vi "Set Channel.vi"(0 "TCS.lvclass in":refnum<class "TCS.lvclass">, 5 "Channel":u8, 7 "I&R In":T1 {"Current" min=0.0}, 11 "error in (no error)":errorcluster) -> (4 "TCS.lvclass out":refnum<class "TCS.lvclass">, 15 "error out":errorcluster)   [LabVIEW 2016, in "TCS.lvclass"]
uses:
  Lib.llb/TCS.lvclass
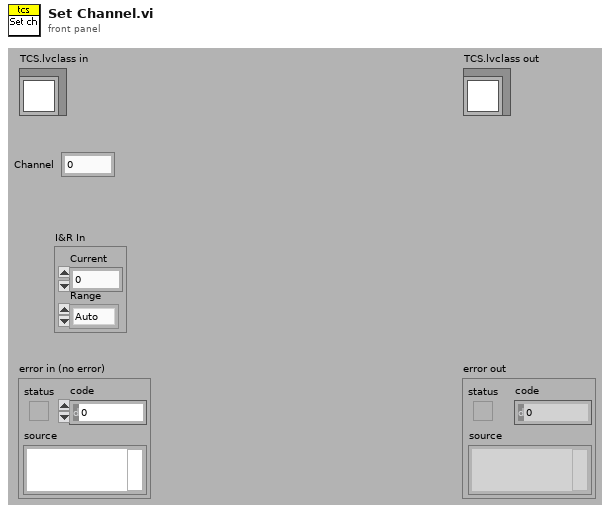
[diagram p1: front panel]
types:
  T1 = cluster{"Current":dbl, "Range":enum8{"Auto", "x1 uA", "x10 uA", "x100 uA", "x1 mA"}}
  T2 = enum8{"Auto", "x1 uA", "x10 uA", "x100 uA", "x1 mA"}
  T3 = cluster{"error":bool, "code":i32, "source":string}
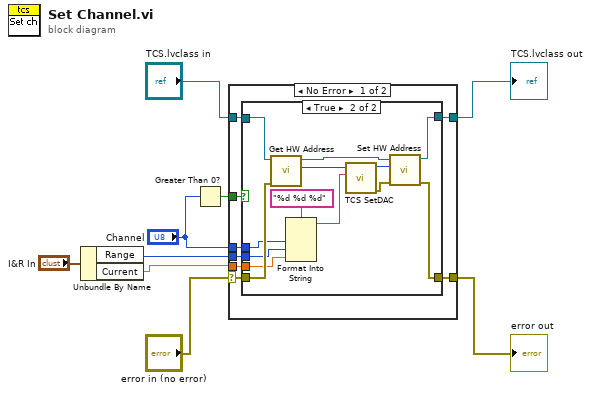
[diagram p0: block diagram]
diagram:
  n1 = Unbundle By Name("I&R In") -> ("Range"=w2:T2, "Current"=w1:dbl)
  n2 = Greater Than 0?(x="Channel") -> (x > 0?=w5:bool)
  n3 = case shown="No Error" "error in (no error)" {
    selector: "error in (no error)" -> [w17 w34]
    tunnel: "TCS.lvclass in" -> [w14 w33]
    tunnel: [w15 w33] -> w8
    tunnel: "Channel" -> [w13 _]
    tunnel: w2 -> [w12 _]
    tunnel: w1 -> [w11 _]
    tunnel: [w16 w34] -> w7
    tunnel: w5 -> [w10 _]
    frame No Error {
      n4 = case shown="True" w10 {
        tunnel: w17 -> [w19 w32]
        tunnel: [w19 w31] -> w16
        tunnel: [w18 w30] -> w15
        tunnel: w14 -> [w18 w29]
        tunnel: w13 -> [_ w23]
        tunnel: w12 -> [_ w22]
        tunnel: w11 -> [_ w21]
        frame False {
          # "Ignore Channel 0"
        }
        frame True {
          n5 = call-dynamic "Get HW Address.vi"("error in (no error)"=w32, "CS.lvclass in"=w29) -> ("HW Address"=w28:i32, "CS.lvclass out"=w20:refnum<class "TCS.lvclass">)  [unwired: 7 in, 1 out]
          n6 = Format Into String(format string="%d %d %d", w23, w22, w21) -> (resulting string=w24:string)  [unwired: 2 in, 1 out]
          n7 = call "TCS SetDAC.vi"("Setup String"=w24, "port number (1:com2)"=w28) -> ("error out"=w25:T3, "port number out"=w27:u8)  [unwired: 4 in]
          n8 = call-dynamic "Set HW Address.vi"("error in (no error)"=w25, "HW Address"=w27, "CS.lvclass in"=w20) -> ("error out"=w31:errorcluster, "CS.lvclass out"=w30:refnum<class "TCS.lvclass">)  [unwired: 7 in]
        }
      }
    }
    frame Error {
    }
  }
  "error out" <- w7
  "TCS.lvclass out" <- w8
